vi "valve_state (SubVI).vi"(10 "Ch. 1 value 2":dbl, 11 "Ch. 1 value":dbl) -> (3 "Boolean":bool)   [LabVIEW 2018]
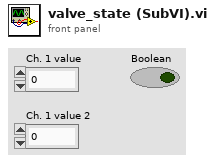
[diagram p1: front panel]
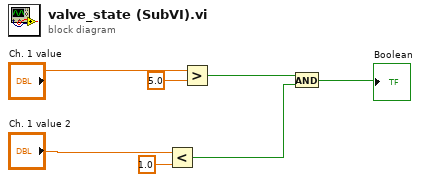
[diagram p0: block diagram]
diagram:
  n1 = Less?(x="Ch. 1 value 2", y=1.0) -> (x < y?=w4:bool)
  n2 = Greater?(x="Ch. 1 value", y=5.0 ("x")) -> (0:w3:bool)
  n3 = And(x=w3, y=w4) -> (x .and. y?=→"Boolean":bool)
